vi "_시리얼_Mark10-설정 (이동속도).vi"(4 "속도(mm/min)":dbl, 5 "시리얼 포트":refnum<visa-resource-name>="COM5") -> (2 "VISA 리소스 이름 출력":refnum<visa-resource-name>)   [LabVIEW 2015]
panel:
  out "전송 문자열":string
  # "MARK10 이동속도 설정"
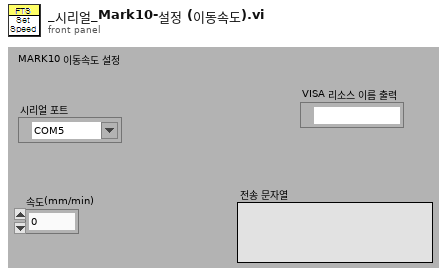
[diagram p1: front panel]
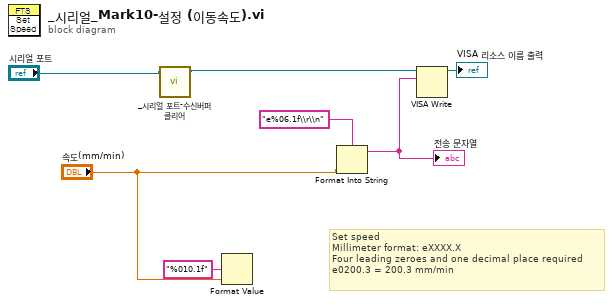
[diagram p0: block diagram]
diagram:
  # "Set speed\nMillimeter format: eXXXX.X\nFour leading zeroes and one decimal place required\ne0200.3 = 200.3 mm/min"
  n1 = call "_시리얼 포트-수신버퍼 클리어.vi"("시리얼 포트"="시리얼 포트") -> ("시리얼 포트 out"=w1:refnum<visa-resource-name>)  [unwired: 3 in, 1 out]
  n2 = Format Value(format string="%010.1f" ("포맷 문자열"), value (0)="속도(mm/min)") -> ()  [unwired: 1 in, 1 out]
  n3 = Format Into String(format string="e%06.1f\\r\\n" ("포맷 문자열"), "속도(mm/min)") -> (resulting string=w6:string)  [unwired: 2 in, 1 out]
  "전송 문자열" <- w6
  n4 = VISA Write(VISA resource name=w1, write buffer=w6) -> (VISA resource name out=→"VISA 리소스 이름 출력":refnum<visa-resource-name>)  [unwired: 1 in, 2 out]
